vi "Read Single Channel U8 1D Array.vi"(8 "error in (no error)":errorcluster, 11 "Model Driver in":refnum<class "Model Driver.lvclass">) -> (0 "error out":errorcluster, 2 "Single Channel U8 1D Array":u8[](array[numeric]), 3 "Model Driver out":refnum<class "Model Driver.lvclass">)   [LabVIEW 2023, in "Model Driver.lvclass"]
uses:
  Model Driver.lvclass
  Model Driver.lvclass/Model Driver.ctl
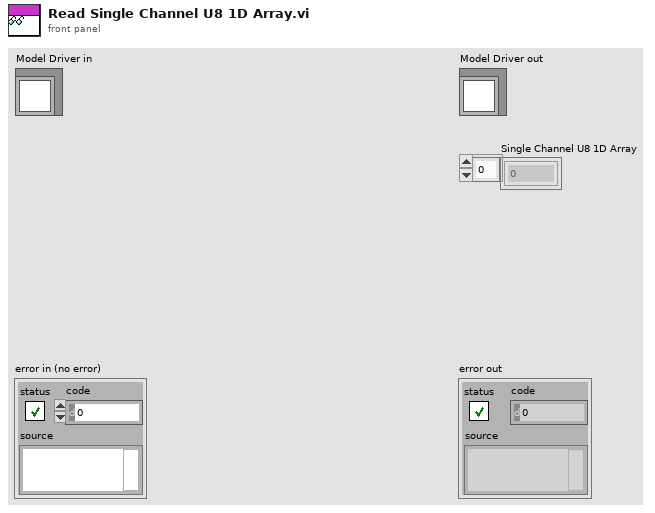
[diagram p1: front panel]
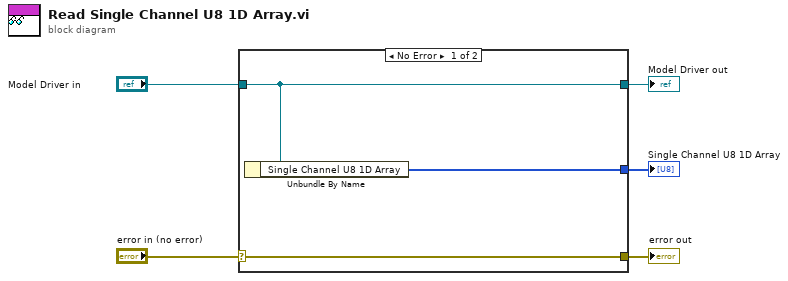
[diagram p0: block diagram]
diagram:
  n1 = case shown="No Error" "error in (no error)" {
    selector: "error in (no error)" -> [w8 w9]
    tunnel: [w8 w9] -> w4
    tunnel: [w7 w10] -> w2
    tunnel: "Model Driver in" -> [w7 w10]
    tunnel: [w6 _] -> w1
    frame No Error {
      n2 = Unbundle By Name(w7) -> ("Single Channel U8 1D Array"=w6:u8[])
    }
    frame Error {
    }
  }
  "error out" <- w4
  "Model Driver out" <- w2
  "Single Channel U8 1D Array" <- w1
